vi "Configure AWGN Power.vi"(8 "error in (no error)":errorcluster, 9 "Power Level (-169.03 dBm)":dbl=-169.03, 10 "Power Control Mode (0: Total)":i32(ring) items=["Total", "Signal", "Noise", "Nchannel"], 11 "VISA resource name":refnum<visa-resource-name>) -> (0 "error out":errorcluster, 3 "VISA resource name out":refnum<visa-resource-name>)   [LabVIEW 2012, in "Agilent PSG MXG Series.lvlib"]
doc: "Configure the power control mode and power level when noise is on.\n\n<B>Notes:</B>\n(1) This VI is valid only in N5172B and N5182B that install <B>Option 660</B>."
uses:
  <instrlib>/Agilent PSG MXG Series/Agilent PSG MXG Series.lvlib
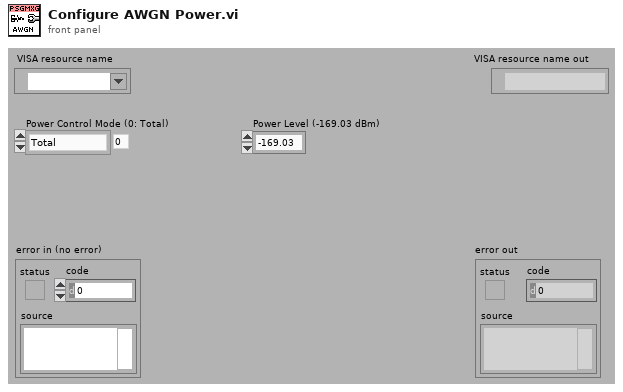
[diagram p1: front panel]
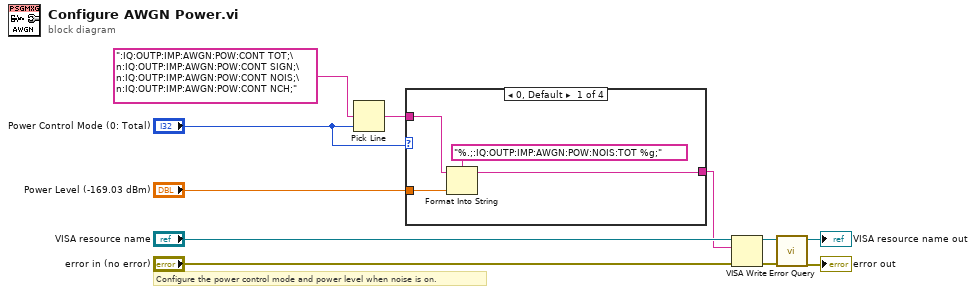
[diagram p0: block diagram]
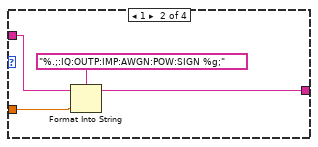
[diagram p2: hidden frame]
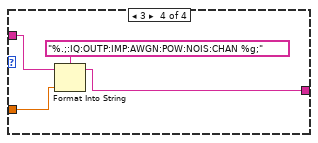
[diagram p4: hidden frame]
diagram:
  # "Configure the power control mode and power level when noise is on."
  n1 = Pick Line(multi-line string=":IQ:OUTP:IMP:AWGN:POW:CONT TOT;\n:IQ:OUTP:IMP:AWGN:POW:CONT SIGN;\n:IQ:OUTP:IMP:AWGN:POW:CONT NOIS;\n:IQ:OUTP:IMP:AWGN:POW:CONT NCH;", line index="Power Control Mode (0: Total)") -> (output string=w10:string)  [unwired: 1 out]
  n2 = case shown="0, Default" "Power Control Mode (0: Total)" {
    tunnel: w10 -> [w14 w19 w20 w24]
    tunnel: "Power Level (-169.03 dBm)" -> [w13 w16 _ w21]
    tunnel: [w12 w17 w20 w22] -> w1
    frame 0, Default {
      n3 = Format Into String(format string="%.;:IQ:OUTP:IMP:AWGN:POW:NOIS:TOT %g;", initial string=w14, w13) -> (resulting string=w12:string)  [unwired: 1 in, 1 out]
    }
    frame 1 {
      n4 = Format Into String(format string="%.;:IQ:OUTP:IMP:AWGN:POW:SIGN %g;", initial string=w19, w16) -> (resulting string=w17:string)  [unwired: 1 in, 1 out]
    }
    frame 2 {
    }
    frame 3 {
      n5 = Format Into String(format string="%.;:IQ:OUTP:IMP:AWGN:POW:NOIS:CHAN %g;", initial string=w24, w21) -> (resulting string=w22:string)  [unwired: 1 in, 1 out]
    }
  }
  n6 = VISA Write(VISA resource name="VISA resource name", write buffer=w1, error in (no error)="error in (no error)") -> (VISA resource name out=w7:refnum<visa-resource-name>, error out=w6:errorcluster)  [unwired: 1 out]
  n7 = call <instrlib>:"Error Query.vi"("error in (no error)"=w6, "VISA resource name"=w7) -> ("error out"=→"error out":errorcluster, "VISA resource name out"=→"VISA resource name out":refnum<visa-resource-name>)  [unwired: 8 out]
